vi "GDSAPI_Example_CreateMethods.vi"() -> ()   [LabVIEW 2020]
uses:
  <resource>/Framework/Providers/Open_GDS/API/GDSAPI_SubVIs/GDSAPI_ClassProviderType.ctl
  <resource>/Framework/Providers/Open_GDS/ClassProviders/Provider_EndevoGOOP300/GOOP300_SubVIs/GOOP300_MethodScopeType.ctl
  <resource>/Framework/Providers/Open_GDS/API/GDSAPI_SubVIs/GDSAPI_MethodType.ctl
  <resource>/Framework/Providers/Open_GDS/ClassProviders/Common/CommonVIs/CommonVIs_AttributeType.ctl
  <resource>/Framework/Providers/Open_GDS/ClassProviders/Common/CommonVIs/CommonVIs_AttributeDataType.ctl
  <resource>/Framework/Providers/Open_GDS/ClassProviders/Common/String/GDSString_AccessScopeModifierType.ctl
  <resource>/Framework/Providers/Open_GDS/API/GDSAPI_CreateClassType.ctl
  <resource>/Framework/Providers/Open_GDS/API/GDSAPI_SubVIs/GDSAPI_ClassTemplateType.ctl
panel:
  out "error out":errorcluster
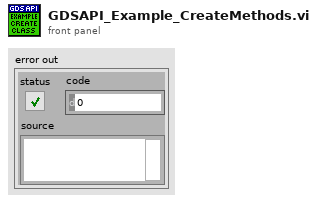
[diagram p1: front panel]
types:
  T1 = typedef "GOOP300_MethodScopeType.ctl" = enum16{"Use Parent Folder Scope", "Public", "Protected", "Private", "Community"}
  T2 = typedef "GDSAPI_MethodType.ctl" = enum16{"Read Attribute", "Write Attribute", "Read & Write Attribute", "None Modifying Method", "Get Property", "Set Property", "Read Property", "Write Property", "Static Method", "Interface Method"}
  T3 = cluster{"MethodName":string, "RelativeMethodPath":path, "MethodDescription":string, "Scope/Visibility":T1, "MethodType":T2, "RelativeProjectClassPath":string, "DynamicDispatchVi":bool, "OverrideMethod(Path)/PropertyMethod(AttributeName)":string}
  T4 = typedef "CommonVIs_AttributeType.ctl" = cluster{"Name":string, "DataType":T5, "ArrayDim":i32, "CtrlPath":path, "DataTypeString":string, "AccessScope":T6, "InitialData":variant}
  T5 = typedef "CommonVIs_AttributeDataType.ctl" = enum16{"UINT8", "INT8", "UINT16", "INT16", "UINT32", "INT32", "UINT64", "INT64", "SGL", "DBL", "EXT", "CSG", "CDB", "CXT", "TimeStamp", "STRING", "PATH", "BOOL", "ENUM", "RefNum", "VIRefNum", "LabVIEW Class", "Cluster", "Variant", "TypeDef", "Waveform", "LabVIEW Object", "Other", "void", "Set", "Map"}
  T6 = typedef "GDSString_AccessScopeModifierType.ctl" = enum16{"public", "private", "protected", "internal"}
  T7 = cluster{"MethodName":string, "RelativeMethodPath":path, "MethodDescription":string, "Scope/Visibility":T1, "MethodType":T2, "RelativeProjectClassPath":string, "DynamicDispatchVi":bool, "OverrideMethod(Path)/PropertyMethod(AttributeName)":string}[]
  T8 = typedef "GDSAPI_ClassProviderType.ctl" = enum16{"LabVIEW Native(By value)", "GOOP-3(By reference)", "GOOP-4(By reference)"}
  T9 = typedef "GDSAPI_CreateClassType.ctl" = cluster{"ClassProvider":T8, "NewClassFolder":path, "ParentLvClassFilePath":path, "ClassName":string, "ClassDescription":string, "ClassTemplate":T10, "ParentInterfacesFilePath":path[]}
  T10 = typedef "GDSAPI_ClassTemplateType.ctl" = enum16{"Standard", "Singleton"}
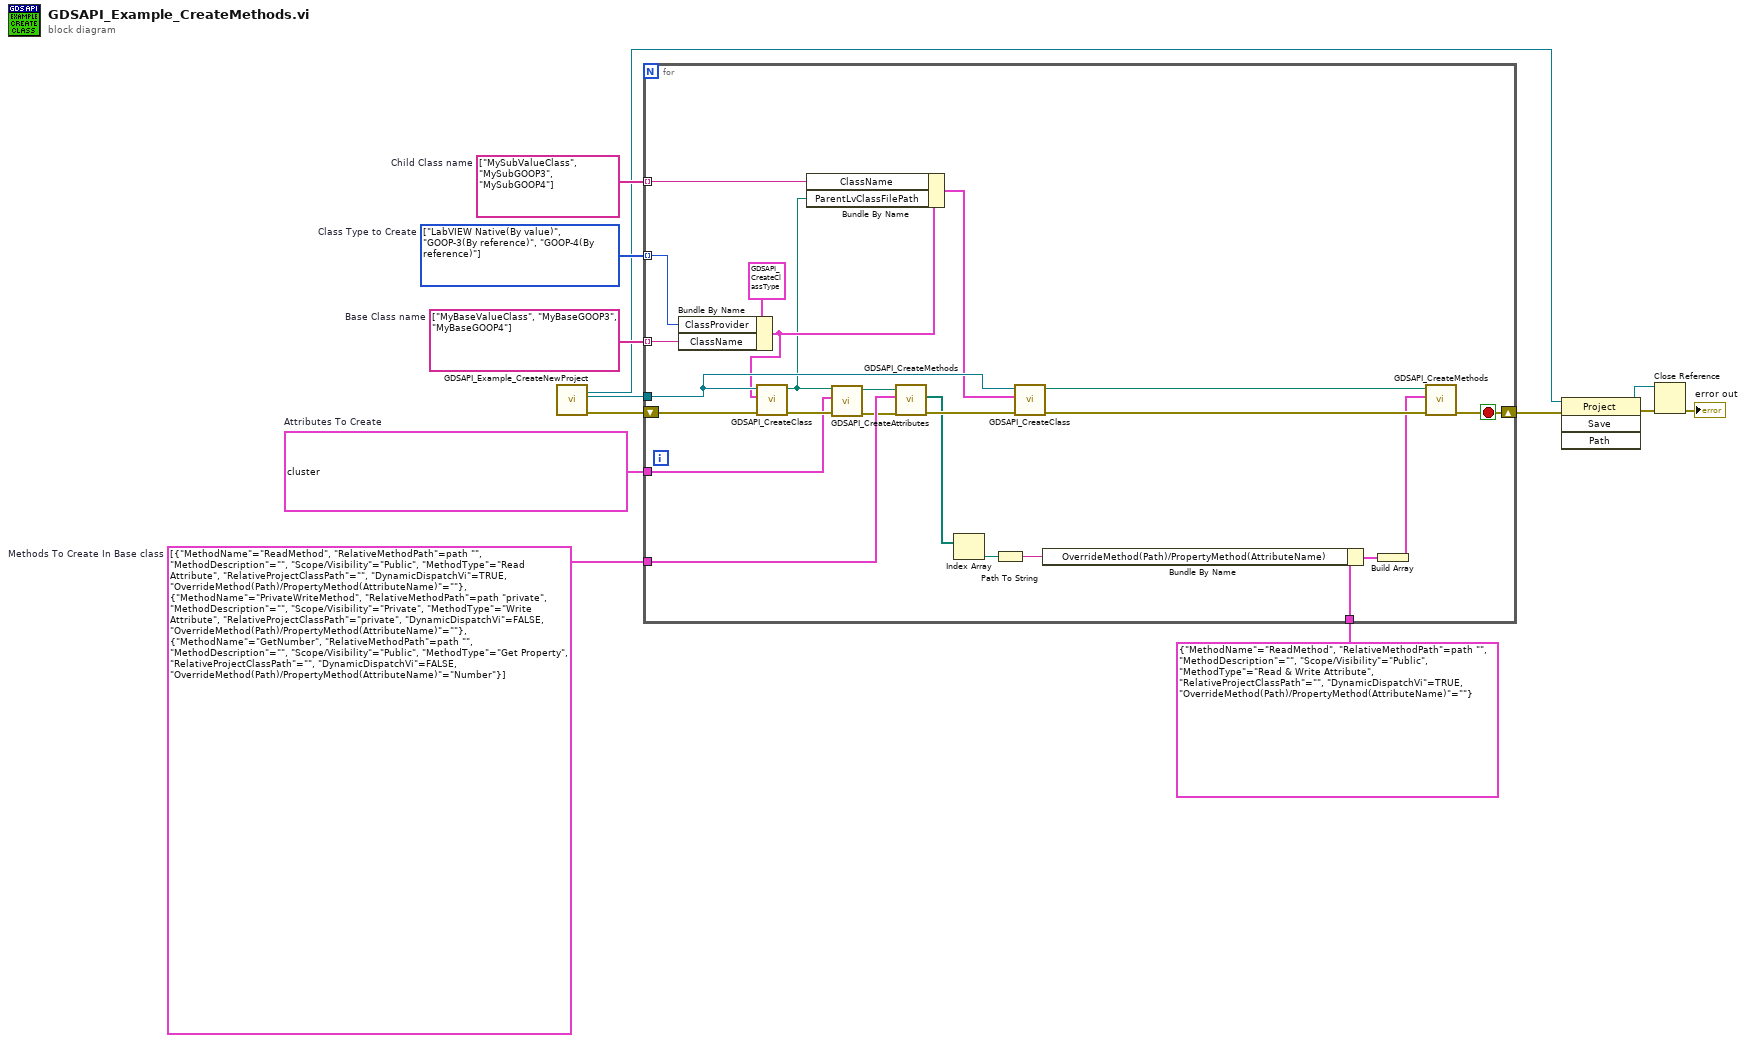
[diagram p0: block diagram]
diagram:
  w2 = T4[] [{"Name"="Number", "DataType"=enum."UINT8", "ArrayDim"=0, "CtrlPath"=path "", "DataTypeString"="", "AccessScope"=enum."public", "InitialData"=variant}, {"Name"="String", "DataType"=enum."STRING", "ArrayDim"=0, "CtrlPath"=path "", "DataTypeString"="", "AccessScope"=enum."public", "InitialData"=variant}, {"Name"="MySelf", "DataType"=enum."LabVIEW Class", "ArrayDim"=0, "CtrlPath"=path "", "DataTypeString"="", "AccessScope"=enum."public", "InitialData"=variant}]  # Attributes To Create
  w4 = T7 [{"MethodName"="ReadMethod", "RelativeMethodPath"=path "", "MethodDescription"="", "Scope/Visibility"=enum."Public", "MethodType"=enum."Read Attribute", "RelativeProjectClassPath"="", "DynamicDispatchVi"=TRUE, "OverrideMethod(Path)/PropertyMethod(AttributeName)"=""}, {"MethodName"="PrivateWriteMethod", "RelativeMethodPath"=path "private", "MethodDescription"="", "Scope/Visibility"=enum."Private", "MethodType"=enum."Write Attribute", "RelativeProjectClassPath"="private", "DynamicDispatchVi"=FALSE, "OverrideMethod(Path)/PropertyMethod(AttributeName)"=""}, {"MethodName"="GetNumber", "RelativeMethodPath"=path "", "MethodDescription"="", "Scope/Visibility"=enum."Public", "MethodType"=enum."Get Property", "RelativeProjectClassPath"="", "DynamicDispatchVi"=FALSE, "OverrideMethod(Path)/PropertyMethod(AttributeName)"="Number"}]  # Methods To Create In Base class
  w9 = string[] ["MySubValueClass", "MySubGOOP3", "MySubGOOP4"]  # Child Class name
  w8 = string[] ["MyBaseValueClass", "MyBaseGOOP3", "MyBaseGOOP4"]  # Base Class name
  w7 = T8[] [enum."LabVIEW Native(By value)", enum."GOOP-3(By reference)", enum."GOOP-4(By reference)"] items=["LabVIEW Native(By value)", "GOOP-3(By reference)", "GOOP-4(By reference)"]  # Class Type to Create
  n1 = call <resource>:"GDSAPI_Example_CreateNewProject.vi"() -> ("error out"=w13:errorcluster, "ProjectItem out"=w12:refnum<vi>, "ProjectRefOut"=w6:refnum<vi>)  [unwired: 8 in, 1 out]
  n2 = for {
    tunnel: w12 -> [w37]
    tunnel: w9 -> [w34] mode=indexing
    tunnel: w8 -> [w33] mode=indexing
    tunnel: w7 -> [w32] mode=indexing
    shift-right: [w26] -> w3
    shift-left: w13 -> [w31]
    tunnel: w4 -> [w29]
    tunnel: w2 -> [w21]
    tunnel: T3 {"MethodName"="ReadMethod", "RelativeMethodPath"=path "", "MethodDescription"="", "Scope/Visibility"=enum."Public", "MethodType"=enum."Read & Write Attribute", "RelativeProjectClassPath"="", "DynamicDispatchVi"=TRUE, "OverrideMethod(Path)/PropertyMethod(AttributeName)"=""} ("CreateMethodData") -> [w17]
    stop <- w26 stop-if-true
    n3 = Bundle By Name(cluster=T9 {"ClassProvider"=enum."LabVIEW Native(By value)", "NewClassFolder"=path "", "ParentLvClassFilePath"=path "", "ClassName"="", "ClassDescription"="", "ClassTemplate"=enum."Standard", "ParentInterfacesFilePath"=[]} ("CreateClassType"), "ClassProvider"=w32, "ClassName"=w33) -> (w35:T9)
    n4 = call <resource>:"GDSAPI_CreateClass.vi"("error in (no error)"=w31, "CreateClassType"=w35, "ProjectItemToCreateClassUnder"=w37) -> ("error out"=w25:errorcluster, "LvClassFileOut"=w23:path)  [unwired: 6 in, 1 out]
    n5 = Bundle By Name(cluster=w35, "ClassName"=w34, "ParentLvClassFilePath"=w23) -> (w36:T9)
    n6 = call <resource>:"GDSAPI_CreateAttributes.vi"("error in (no error)"=w25, "Attributes"=w21, "ClassPath(*.lvclass)"=w23) -> ("error out"=w24:errorcluster, "ClassPathOut(*.lvclass)"=w22:path)  [unwired: 7 in]
    n7 = call <resource>:"GDSAPI_CreateMethods.vi"("error in (no error)"=w24, "Methods"=w29, "ClassPath(*.lvclass)"=w22) -> ("error out"=w30:errorcluster, "MethodPath"=w19:path[])  [unwired: 6 in, 1 out]
    n8 = Index Array(array=w19) -> (element=w18:path)  [unwired: 1 in]
    n9 = Path To String(path=w18) -> (string=w16:string)
    n10 = call <resource>:"GDSAPI_CreateClass.vi"("error in (no error)"=w30, "CreateClassType"=w36, "ProjectItemToCreateClassUnder"=w37) -> ("error out"=w28:errorcluster, "LvClassFileOut"=w27:path)  [unwired: 6 in, 1 out]
    n11 = Bundle By Name(cluster=w17, "OverrideMethod(Path)/PropertyMethod(AttributeName)"=w16) -> (w15:T3)
    n12 = Build Array(w15) -> (w14:T7)
    n13 = call <resource>:"GDSAPI_CreateMethods.vi"("error in (no error)"=w28, "Methods"=w14, "ClassPath(*.lvclass)"=w27) -> ("error out"=w26:errorcluster)  [unwired: 6 in, 2 out]
  }
  n14 = invoke class="Project" method="Save"(reference=w6, error in=w3) -> (reference out=w10:refnum<vi>, error out=w11:errorcluster)  [unwired: 2 in, 2 out]
  n15 = Close Reference(reference=w10, error in (no error)=w11) -> (error out=→"error out":errorcluster)
